vi "setUp.vi"(8 "error in (no error)":errorcluster, 11 "reference in":refnum<class "testcase-CSMAttributes.lvclass">) -> (0 "error out":errorcluster, 3 "reference out":refnum<class "testcase-CSMAttributes.lvclass">)   [LabVIEW 2017, in "testcase-CSMAttributes.lvclass"]
doc: "setUp runs prior to the test method during test execution. Use this method to initialize any object data required by your tests."
uses:
  testcase-CSMAttributes.lvclass
  C:/Program Files (x86)/National Instruments/LabVIEW 2017/vi.lib/addons/_JKI Toolkits/VI Tester/TestCase.llb/TestCase.lvclass
  testcase-CSMAttributes.lvclass/testcase-CSMAttributes.ctl
  <vilib>/addons/_JKI Toolkits/VI Tester/TestCase.llb/TestCase.lvclass
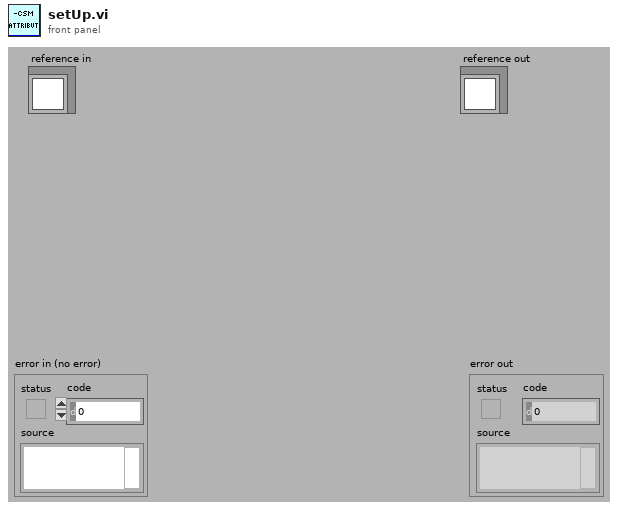
[diagram p1: front panel]
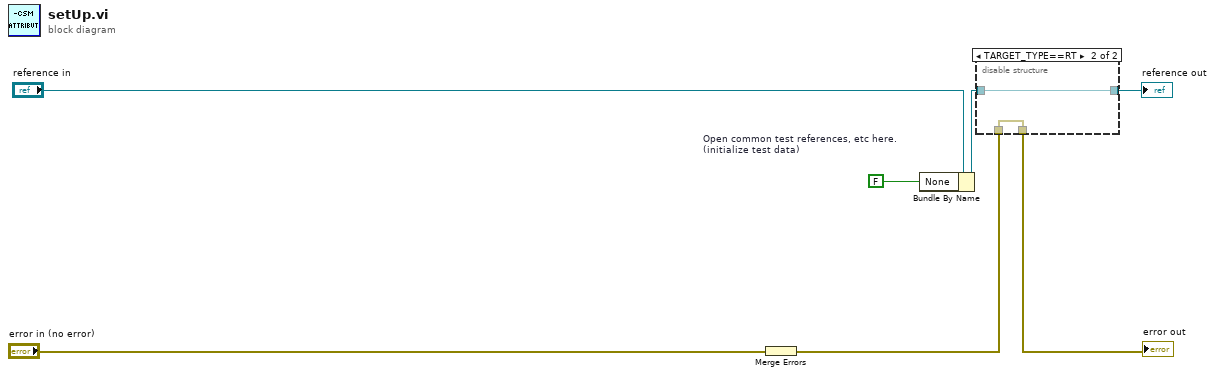
[diagram p0: block diagram]
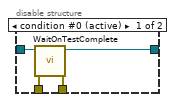
[diagram p2: hidden frame]
diagram:
  w2 = FALSE  # Open common test references, etc here. (initialize test data)
  n1 = Merge Errors("error in (no error)") -> (w1:errorcluster)
  n2 = Bundle By Name(cluster="reference in", "None"=w2) -> (w3:refnum<class "testcase-CSMAttributes.lvclass">)
  n3 = disable-structure shown="TARGET_TYPE==RT" {
    disable-tunnel: w1 -> [w11 w12]
    disable-tunnel: [w10 w12] -> w6
    disable-tunnel: [w9 w13] -> w4
    disable-tunnel: w3 -> [w8 w13]
    frame condition #0 (active) {
      n4 = call <vilib>:"WaitOnTestComplete.vi"("error in (no error)"=w11, "TestCase in"=w8) -> ("error out"=w10:errorcluster, "TestCase out"=w9:refnum<class "testcase-CSMAttributes.lvclass">)  [unwired: 8 in]
    }
    frame condition #1 {
    }
  }
  "error out" <- w6
  "reference out" <- w4
